vi "-8780 ReadRate not set--error.vi"(8 "error in":errorcluster) -> (0 "error out":errorcluster)   [LabVIEW 2024, in "Communicator Worker.lvlib" / "Communicator Worker.lvclass"]
uses:
  Communicator Worker.lvclass
  Communicator Worker.lvclass/Communicator Worker.ctl
  Common-LabVIEW-Helpers/Source/Error Helpers.lvlib
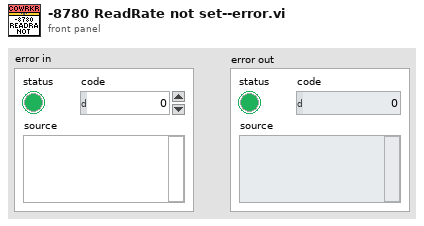
[diagram p1: front panel]
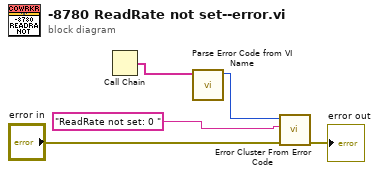
[diagram p0: block diagram]
diagram:
  n1 = Call Chain() -> (call chain=w2:string[])
  n2 = call "Parse Error Code from VI Name.vi"("Call Chain"=w2) -> ("Error Code"=w1:i32)  [unwired: 10 in]
  n3 = call <vilib>:"Error Cluster From Error Code.vi"("error in (no error)"="error in", "error message (\"\")"="ReadRate not set: 0 " ("error message (\"\")"), "error code (0)"=w1) -> ("error out"=→"error out":errorcluster)  [unwired: 6 in]
